vi "configuration UI.vi"() -> ()   [LabVIEW 2013, in "user tag bus module editor node.lvclass"]
uses:
  user tag bus module editor node.lvclass
  <vilib>/CEF_TreeControl/Node/NodeRef.ctl
  <vilib>/CEF_TreeControl/Node/NISE_CEF_Node.lvclass
  <vilib>/NI/AMC/Message Queue.ctl
  <vilib>/NI/AMC/Message.ctl
  <vilib>/NI/Tools/Keyed Array/KeyedArray.ctl
  <vilib>/CEF_TreeControl/Node/UserEventRef.ctl
  <vilib>/CEF_TreeControl/Controls/EventCluster.ctl
  module/configuration/user tag bus module configuration.lvclass
  module/configuration/control module configuration.ctl
  <vilib>/NI/Tag Bus Module Framework/channel/TBM channel.lvclass
  module/configuration/gains.ctl
  module/configuration/state module configuration.ctl
  user tag bus module editor node.lvclass/user tag bus module editor node.ctl
  <vilib>/NI/Tag Bus Module Framework/root configuration/TBM configuration.lvclass/TBM configuration.ctl
  Configuration Editor/Classes/Engine Parent/Engine Parent Editor Node.lvclass
  module/configuration/user tag bus module configuration.lvclass/user tag bus module configuration.ctl
  Read sort_.vi
  module/configuration/Read state module configuration.vi
  Write sort_.vi
  <vilib>/NI/Tag Bus Module Framework/root configuration/Read instance name.vi
  Configuration Editor/Classes/Module editor node/Read Module Configuration.vi
  <vilib>/NI/Tag Bus Module Framework/root configuration/create GUID.vi
  <vilib>/NI/Tag Bus Module Framework/module configuration/TBM module configuration.lvclass
  <vilib>/CEF_TreeControl/NISE_CEF_TreeControl.lvlib
  <vilib>/NI/Tools/Keyed Array/Tools_KeyedArray.lvlib
  <vilib>/NI/AMC/AMC.lvlib
panel:
  in  "Tab Control":T1(tab)
  in  "delete":bool
  in  "add":bool
  in  "Result Tag":u16(ring)
  in  "PV Tag":u16(ring)
  in  "Setpoint Tag":u16(ring)
  in  "Functions":i32(listbox)
  in  "Function Name":string
  in  "Lower Limit":dbl=-100.0
  in  "Upper Limit":dbl=100.0
  in  "Ki":dbl
  in  "Kd":dbl
  in  "Kp":dbl
  in  "Output Tag":u16(ring)
  in  "Input Tag":u16(ring)
  in  "Initial State":u8
  in  "user event":T2
  in  "main queue":T3
  in  "node ref":T4
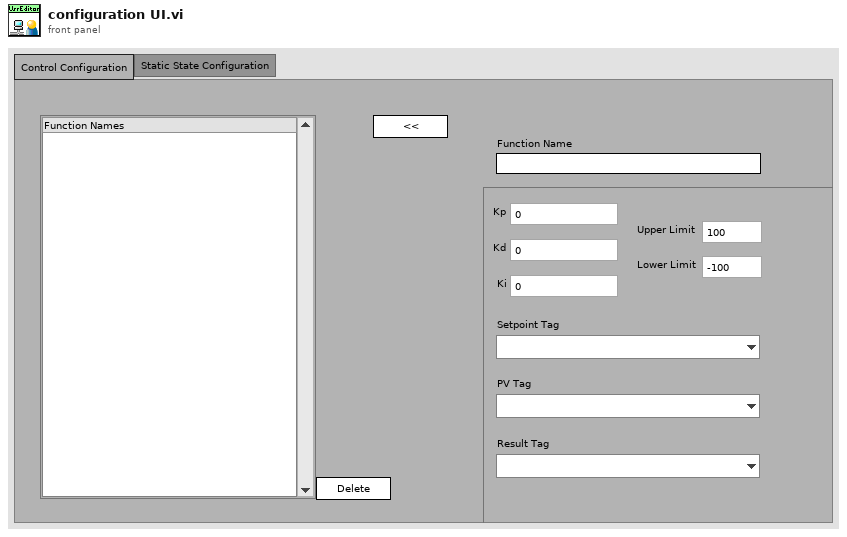
[diagram p1: front panel]
types:
  T1 = enum32{"Control Configuration", "Static State Configuration"}
  T2 = typedef "NISE_CEF_Node.lvclass/UserEventRef.ctl" = refnum<user-event>
  T3 = typedef "AMC.lvlib/Message Queue.ctl" = refnum<queue>
  T4 = typedef "NISE_CEF_Node.lvclass/NodeRef.ctl" = refnum<data-value>
  T5 = typedef "user tag bus module configuration.lvclass/state module configuration.ctl" = cluster{"fixed input":refnum<class "TBM channel.lvclass">, "fixed output":refnum<class "TBM channel.lvclass">, "initial state":u8}
  T6 = typedef "user tag bus module configuration.lvclass/control module configuration.ctl" = cluster{"name":string, "setpoint":refnum<class "TBM channel.lvclass">, "process variable":refnum<class "TBM channel.lvclass">, "output":refnum<class "TBM channel.lvclass">, "gains":T7, "output range":cluster{"output high":dbl, "output low":dbl}}
  T7 = typedef "user tag bus module configuration.lvclass/gains.ctl" = cluster{"Kp":dbl, "Ki":dbl, "Kd":dbl}
  T8 = typedef "NISE_CEF_TreeControl.lvlib/EventCluster.ctl" = cluster{"command":string, "data":string}
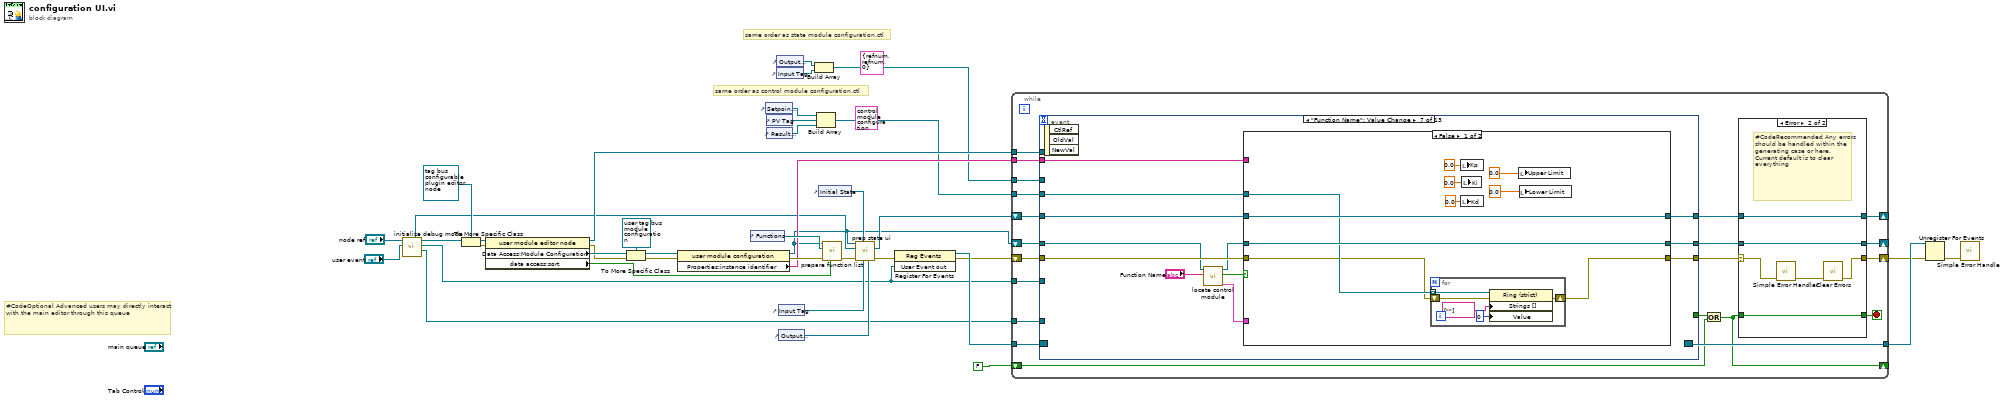
[diagram p0: block diagram]
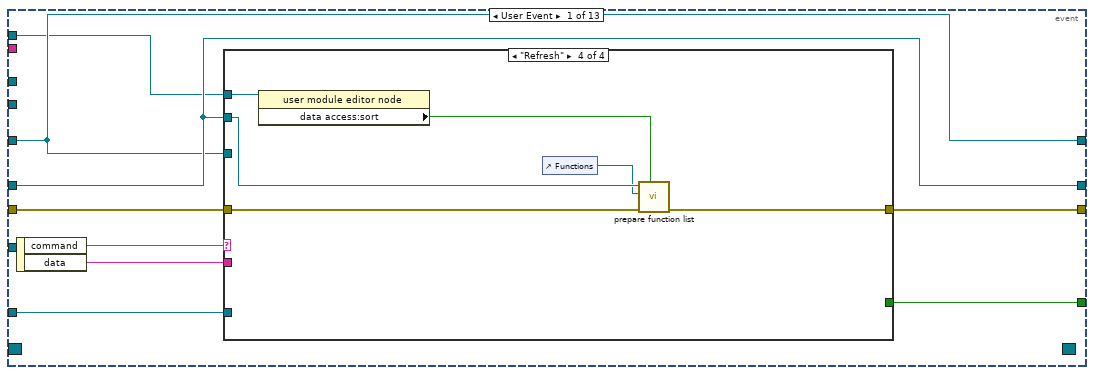
[diagram p3: hidden frame]
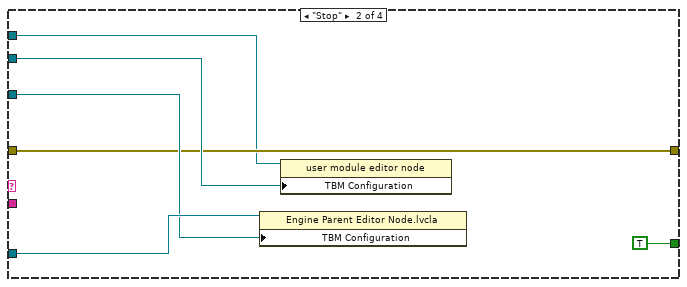
[diagram p5: hidden frame]
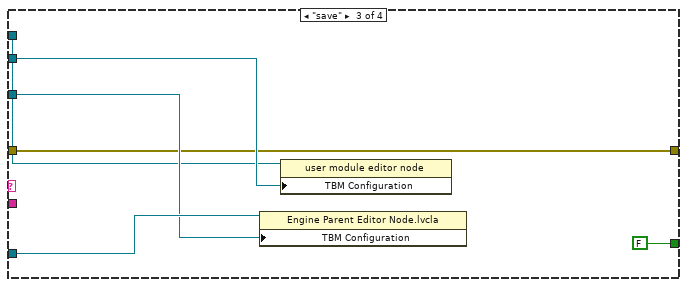
[diagram p6: hidden frame]
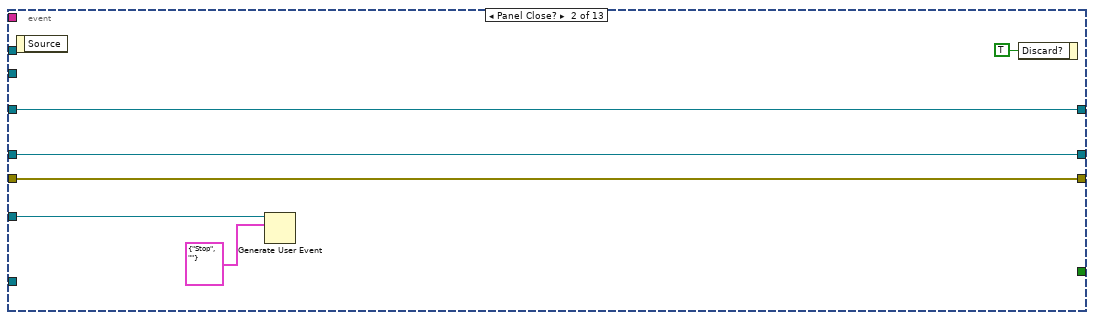
[diagram p7: hidden frame]
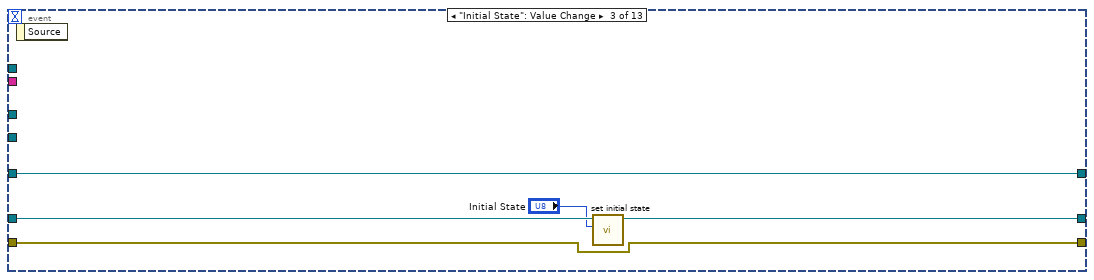
[diagram p8: hidden frame]
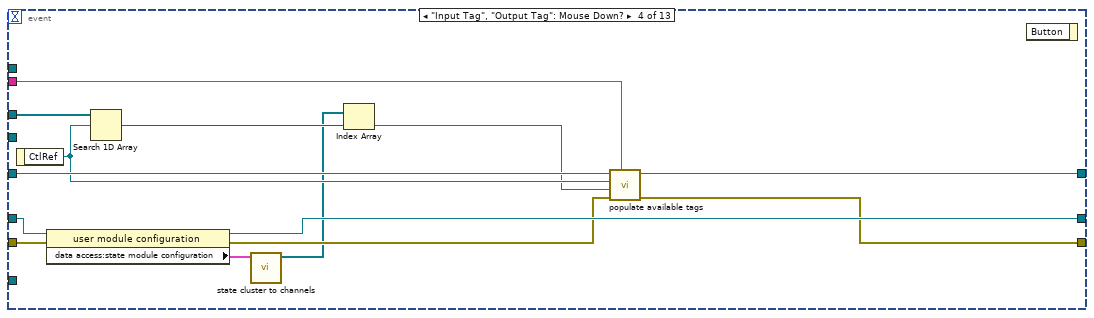
[diagram p9: hidden frame]
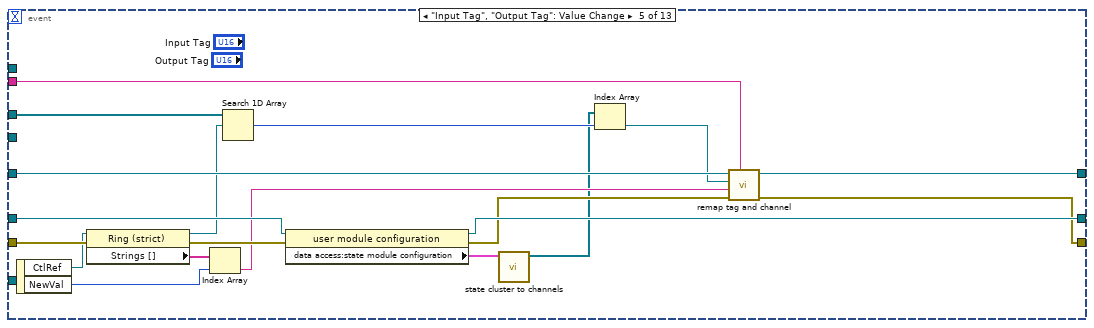
[diagram p10: hidden frame]
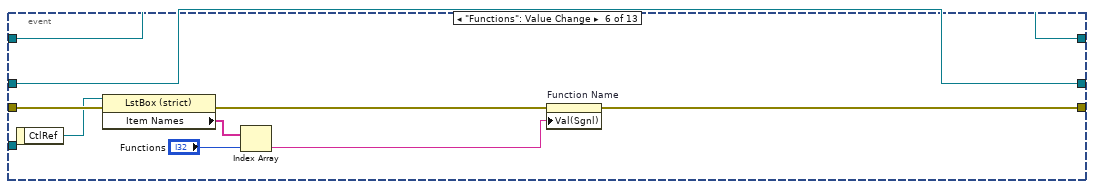
[diagram p11: hidden frame]
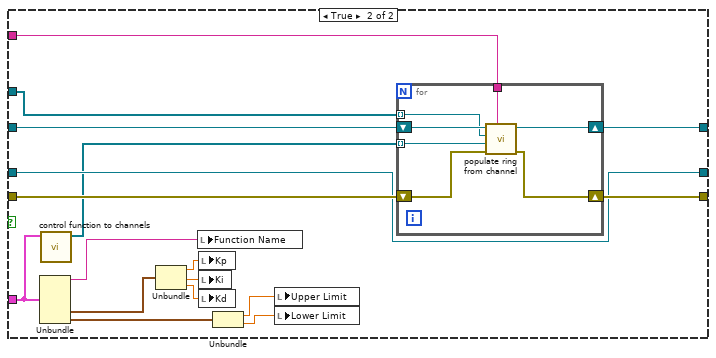
[diagram p12: hidden frame]
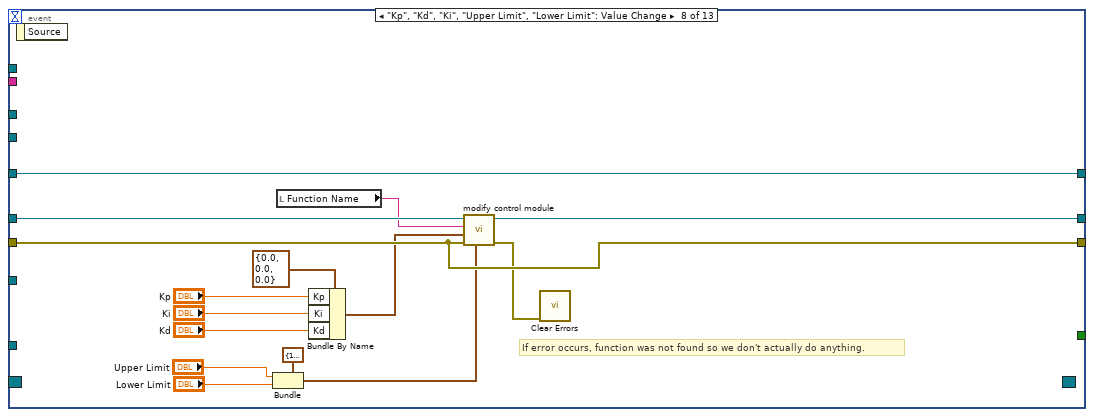
[diagram p13: hidden frame]
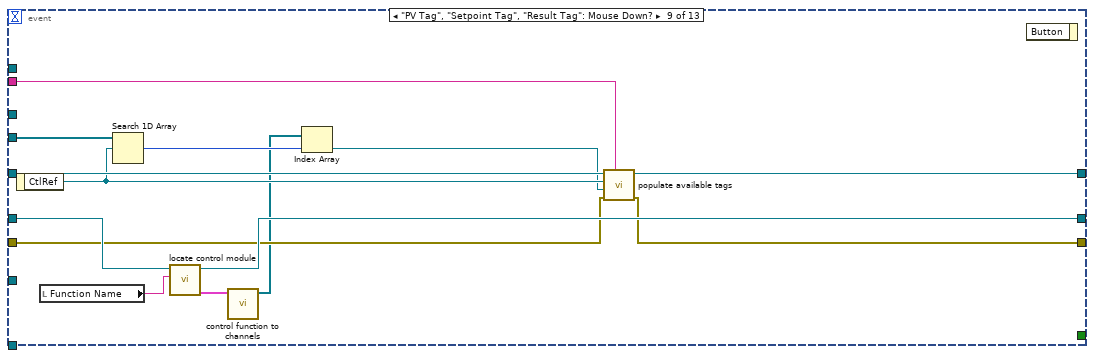
[diagram p14: hidden frame]
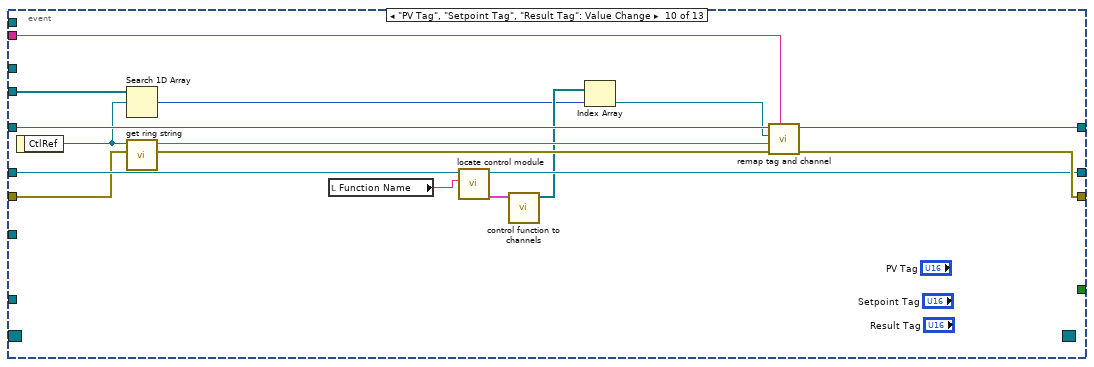
[diagram p15: hidden frame]
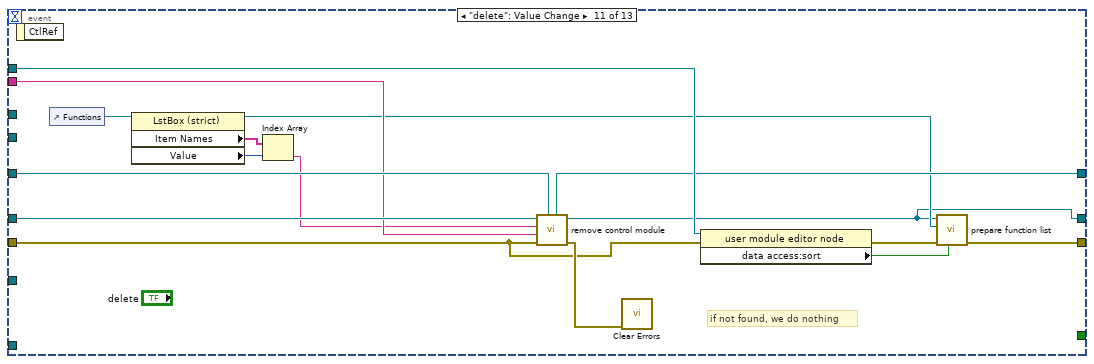
[diagram p16: hidden frame]
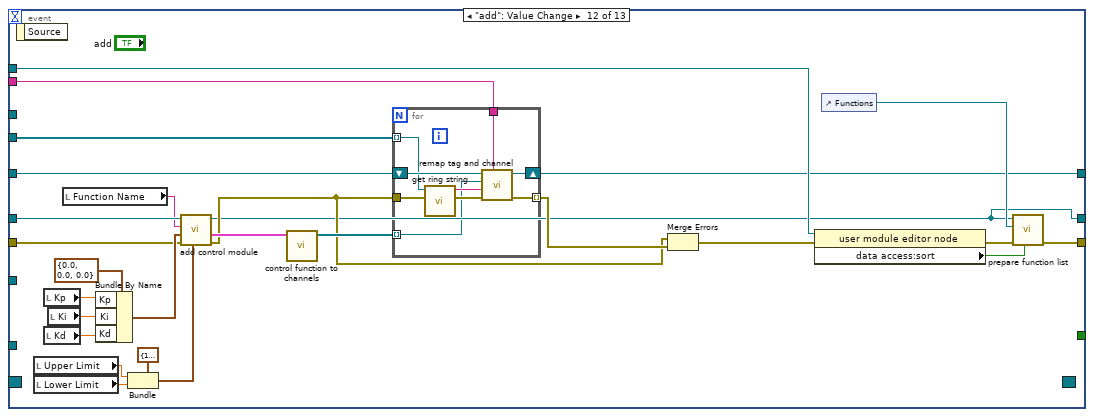
[diagram p17: hidden frame]
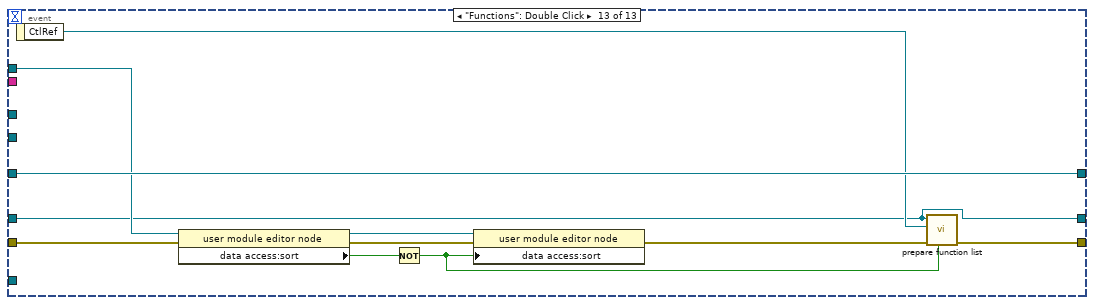
[diagram p18: hidden frame]
diagram:
  (unwired) T5 {"fixed input"=refnum, "fixed output"=refnum, "initial state"=0} ("state module configuration")
  (unwired) T6 {"name"="", "setpoint"=refnum, "process variable"=refnum, "output"=refnum, "gains"={"Kp"=0.0, "Ki"=0.0, "Kd"=0.0}, "output range"={"output high"=100.0, "output low"=-100.0}} ("control module configuration")
  # "same order as control module configuration.ctl"
  # "same order as state module configuration.ctl"
  # "#CodeOptional Advanced users may directly interact with the main editor through this queue"
  n1 = call "initialize debug mode.vi"("User Event in"="user event", "editor node in"="node ref") -> ("engine"=w11:refnum<data-value>, "User Event out"=w4:T2, "editor node out"=w14:T4, "Engine Configuration"=w10:refnum<class "engine configuration.lvclass">)  [unwired: 6 in]
  n2 = To More Specific Class(target class=refnum<data-value> refnum ("data value reference"), reference=w14) -> (specific class reference=w32:refnum<data-value>, error out=w31:errorcluster)  [unwired: 1 in]
  n3 = property class="user module editor node"(reference=w32, error in=w31) -> (reference out=w16:refnum<data-value>, error out=w26:errorcluster, "Data Access:Module Configuration"=w30:refnum<class "TBM module configuration.lvclass">, "data access:sort"=w15:bool)
  n4 = To More Specific Class(target class=refnum<class "user tag bus module configuration.lvclass"> refnum ("user module configuration"), reference=w30, error in=w26) -> (specific class reference=w24:refnum<class "user tag bus module configuration.lvclass">, error out=w28:errorcluster)
  n5 = property class="user module configuration"(reference=w24, error in=w28) -> (reference out=w3:refnum<class "user tag bus module configuration.lvclass">, error out=w25:errorcluster, "Properties:instance identifier"=w23:string)
  n6 = control-ref of="Functions"() -> (w27:refnum<vi>)
  n7 = control-ref of="Setpoint Tag"() -> (w2:refnum<vi>)
  n8 = control-ref of="PV Tag"() -> (w7:refnum<vi>)
  n9 = control-ref of="Result Tag"() -> (w1:refnum<vi>)
  n10 = control-ref of="Output Tag"() -> (w8:refnum<vi>)
  n11 = control-ref of="Input Tag"() -> (w9:refnum<vi>)
  n12 = control-ref of="Input Tag"() -> (w19:refnum<vi>)
  n13 = control-ref of="Output Tag"() -> (w18:refnum<vi>)
  n14 = Build Array(w8, w9) -> (w6:refnum<vi>[])
  n15 = Build Array(w2, w7, w1) -> (w5:refnum<vi>[])
  n16 = control-ref of="Initial State"() -> (w20:refnum<vi>)
  n17 = call "prepare function list.vi"("sort?"=w15, "error in"=w25, "Functions listbox"=w27, "configuration in"=w3) -> ("error out"=w21:errorcluster)  [unwired: 5 in]
  n18 = call "prep state ui.vi"("Output Tag"=w18, "Input Tag"=w19, "Initial State"=w20, "error in"=w21, "engine configuration in"=w10, "user tag bus module configuration in"=w3) -> ("error out"=w22:errorcluster, "engine configuration out"=w17:refnum<class "engine configuration.lvclass">)  [unwired: 4 in]
  n19 = register-events(error in=w22, w4) -> (reference out=w39:refnum<event-registration>, error out=w34:errorcluster)  [unwired: 1 in]
  n20 = while {
    tunnel: w39 -> [w60]
    tunnel: [w59] -> w38
    shift-right: [w52] -> w37
    shift-left: w34 -> [w58]
    shift-right: [w54] -> _
    shift-left: FALSE -> [w53]
    shift-right: [w49] -> _
    shift-left: w3 -> [w51]
    shift-right: [w46] -> _
    shift-left: w17 -> [w48]
    tunnel: w23 -> [w45]
    tunnel: w16 -> [w44]
    tunnel: w11 -> [w43]
    tunnel: w6 -> [w42]
    tunnel: w5 -> [w41]
    tunnel: w4 -> [w40]
    stop <- w56 stop-if-true
    n21 = event shown="[6] \"Function Name\": Value Change" {
      selector: w60 -> [_ _ _ _ _ _ _ _ _ _ _ _ _]
      dyn-events: [_ _ _ _ _ _ _ _ _ _ _ _ _] -> w59
      timeout: _ -> [_ _ _ _ _ _ _ _ _ _ _ _ _]
      tunnel: [w77 _ _ _ _ _ _ _ _ _ _ _ _] -> w55
      tunnel: [w78 w104 w108 w119 w134 w143 w159 w216 w224 w245 w261 w290 w309] -> w57
      tunnel: w58 -> [w79 w104 w108 w123 w142 w151 w163 w216 w225 w238 w258 w272 w308]
      tunnel: [w75 w103 w107 w120 w136 w150 w160 w214 w230 w241 w248 w264 w300] -> w50
      tunnel: w51 -> [w75 w103 w109 w121 w137 w150 w158 w217 w231 w242 w263 w282 w300]
      tunnel: w48 -> [w74 w102 w105 w118 w139 w149 w161 w212 w228 w247 w255 w283 w310]
      tunnel: [w74 w102 w105 w122 w135 w149 w162 w212 w227 w246 w254 w284 w310] -> w47
      tunnel: w45 -> [_ _ _ w117 w132 _ w154 _ w226 w244 w253 w285 _]
      tunnel: w44 -> [w73 _ _ _ _ _ _ _ _ _ w256 w286 w304]
      tunnel: w43 -> [w72 _ _ _ _ _ _ _ _ _ _ _ _]
      tunnel: w42 -> [_ _ _ w115 w130 _ _ _ _ _ _ _ _]
      tunnel: w41 -> [_ _ _ _ _ _ w152 _ w222 w237 _ w267 _]
      tunnel: w40 -> [_ w100 _ _ _ _ _ _ _ _ _ _ _]
      event User Event {
        n22 = event-data() -> ("command"=w76:string, "data"=w71:string)  [unwired: 1 in]
        n23 = case shown="\"Refresh\"" w76 {
          tunnel: [_ TRUE FALSE _] -> w77
          tunnel: w72 -> [_ w85 w91 _]
          tunnel: w75 -> [_ w84 w90 w95]
          tunnel: w74 -> [_ w83 w89 _]
          tunnel: w79 -> [w80 w82 w88 w96]
          tunnel: [w80 w82 w88 w97] -> w78
          tunnel: w73 -> [_ w81 w87 w98]
          tunnel: w71 -> [_ _ _ _]
          frame Default {
          }
          frame "Stop" {
            n24 = property class="Engine Parent Editor Node.lvcla"(reference=w85, "TBM Configuration"=w83) -> ()  [unwired: 1 in, 2 out]
            n25 = property class="user module editor node"(reference=w81, "TBM Configuration"=w84) -> ()  [unwired: 1 in, 2 out]
          }
          frame "save" {
            n26 = property class="Engine Parent Editor Node.lvcla"(reference=w91, "TBM Configuration"=w89) -> ()  [unwired: 1 in, 2 out]
            n27 = property class="user module editor node"(reference=w87, "TBM Configuration"=w90) -> ()  [unwired: 1 in, 2 out]
          }
          frame "Refresh" {
            n28 = property class="user module editor node"(reference=w98) -> ("data access:sort"=w94:bool)  [unwired: 1 in, 2 out]
            n29 = control-ref of="Functions"() -> (w93:refnum<vi>)
            n30 = call "prepare function list.vi"("sort?"=w94, "error in"=w96, "Functions listbox"=w93, "configuration in"=w95) -> ("error out"=w97:errorcluster)  [unwired: 5 in]
          }
        }
      }
      event Panel Close? {
        n31 = event-data() -> ()  [unwired: 1 in, 1 out]
        n32 = Generate User Event(user event=w100, event data cluster=T8 {"command"="Stop", "data"=""} ("event data")) -> ()  [unwired: 2 in, 2 out]
        n33 = event-data("Discard?"=TRUE) -> ()  [unwired: 1 in, 1 out]
      }
      event "Initial State": Value Change {
        n34 = event-data() -> ()  [unwired: 1 in, 1 out]
        n35 = call "set initial state.vi"("state module configuration.initial state"="Initial State", "tag bus configurable plugin module configuration in"=w109) -> ("tag bus configurable plugin module configuration out"=w107:refnum<class "user tag bus module configuration.lvclass">)  [unwired: 9 in]
      }
      event "Input Tag", "Output Tag": Mouse Down? {
        n36 = event-data() -> ("CtlRef"=w114:refnum<vi>)  [unwired: 1 in]
        n37 = property class="user module configuration"(reference=w121, error in=w123) -> (reference out=w120:refnum<class "user tag bus module configuration.lvclass">, error out=w116:errorcluster, "data access:state module configuration"=w112:T5)
        n38 = Search 1D Array(1D array=w115, element=w114) -> (index of element=w113:i32)  [unwired: 1 in]
        n39 = call "state cluster to channels.vi"("state module configuration"=w112) -> ("channels"=w111:refnum<class "TBM channel.lvclass">[])  [unwired: 10 in]
        n40 = Index Array(array=w111, index=w113) -> (element=w110:refnum<class "TBM channel.lvclass">)
        n41 = call "populate available tags.vi"("instance id"=w117, "error in"=w116, "channel"=w110, "CtlRef"=w114, "engine configuration in"=w118) -> ("error out"=w119:errorcluster, "engine configuration out"=w122:refnum<class "engine configuration.lvclass">)  [unwired: 5 in]
        n42 = event-data() -> ()  [unwired: 2 in, 1 out]
      }
      event "Input Tag", "Output Tag": Value Change {
        n43 = event-data() -> ("CtlRef"=w141:refnum<vi>, "NewVal"=w128:u16)  [unwired: 1 in]
        n44 = property on="Property Node" class="Ring (strict)"(reference=w141, error in=w142) -> (reference out=w129:refnum<vi>, error out=w138:errorcluster, "Strings []"=w140:string[])
        n45 = Index Array(array=w140, index=w128) -> (element=w131:string)
        n46 = Search 1D Array(1D array=w130, element=w129) -> (index of element=w126:i32)  [unwired: 1 in]
        n47 = property class="user module configuration"(reference=w137, error in=w138) -> (reference out=w136:refnum<class "user tag bus module configuration.lvclass">, error out=w133:errorcluster, "data access:state module configuration"=w127:T5)
        n48 = call "state cluster to channels.vi"("state module configuration"=w127) -> ("channels"=w125:refnum<class "TBM channel.lvclass">[])  [unwired: 10 in]
        n49 = Index Array(array=w125, index=w126) -> (element=w124:refnum<class "TBM channel.lvclass">)
        n50 = call "remap tag and channel.vi"("instance id"=w132, "error in"=w133, "tag name"=w131, "channel"=w124, "engine configuration in"=w139) -> ("error out"=w134:errorcluster, "engine configuration out"=w135:refnum<class "engine configuration.lvclass">)  [unwired: 5 in]
      }
      event "Functions": Value Change {
        n51 = event-data() -> ("CtlRef"=w148:refnum<vi>)  [unwired: 1 in]
        n52 = property class="LstBox (strict)"(reference=w148, error in=w151) -> (error out=w144:errorcluster, "Item Names"=w147:string[])  [unwired: 1 out]
        n53 = Index Array(array=w147, index="Functions") -> (element=w145:string)
        n54 = property on="Function Name" class="Str"(error in=w144, "Val(Sgnl)"=w145) -> (error out=w143:errorcluster)  [unwired: 1 in, 1 out]
      }
      event "Function Name": Value Change {
        n55 = event-data() -> ()  [unwired: 1 in, 3 out]
        n56 = call "locate control module.vi"("name"="Function Name", "user module configuration in"=w158) -> ("module duplicate"=w155:T6, "found"=w156:bool, "user module configuration out"=w157:refnum<class "user tag bus module configuration.lvclass">)  [unwired: 6 in, 1 out]
        n57 = case shown="False" w156 {
          tunnel: [w173 w187] -> w162
          tunnel: w161 -> [w173 w185]
          tunnel: w157 -> [w172 w182]
          tunnel: [w172 w182] -> w160
          tunnel: w163 -> [w170 w184]
          tunnel: [w169 w183] -> w159
          tunnel: w155 -> [_ w181]
          tunnel: w154 -> [_ w186]
          tunnel: w152 -> [w171 w180]
          frame False {
            n58 = for {
              shift-right: [w178] -> w169
              shift-left: w170 -> [w177]
              tunnel: w171 -> [w175] mode=indexing
              n59 = property on="Property Node" class="Ring (strict)"(reference=w175, error in=w177, "Strings []"=string[] [""], "Value"=u16 0) -> (error out=w178:errorcluster)  [unwired: 1 out]
            }
            n60 = local write "Kp"(0.0 ("Kp")) -> ()
            n61 = local write "Kd"(0.0 ("Kp")) -> ()
            n62 = local write "Ki"(0.0 ("Kp")) -> ()
            n63 = local write "Upper Limit"(0.0 ("Kp")) -> ()
            n64 = local write "Lower Limit"(0.0 ("Kp")) -> ()
          }
          frame True {
            n65 = Unbundle(w181) -> ("name"=w188:string, "gains"=w195:T7, "output range"=w194:cluster{"output high":dbl, "output low":dbl})  [unwired: 3 out]
            n66 = call "control function to channels.vi"("control module configuration"=w181) -> ("channels"=w179:refnum<class "TBM channel.lvclass">[])  [unwired: 10 in]
            n67 = Unbundle(w195) -> ("Kp"=w189:dbl, "Ki"=w190:dbl, "Kd"=w191:dbl)
            n68 = local write "Function Name"(w188) -> ()
            n69 = local write "Kp"(w189) -> ()
            n70 = local write "Ki"(w190) -> ()
            n71 = local write "Kd"(w191) -> ()
            n72 = Unbundle(w194) -> ("output high"=w192:dbl, "output low"=w193:dbl)
            n73 = local write "Upper Limit"(w192) -> ()
            n74 = local write "Lower Limit"(w193) -> ()
            n75 = for {
              tunnel: w186 -> [w201]
              shift-right: [w202] -> w187
              shift-left: w185 -> [w200]
              shift-right: [w198] -> w183
              shift-left: w184 -> [w199]
              tunnel: w180 -> [w197] mode=indexing
              tunnel: w179 -> [w196] mode=indexing
              n76 = call "populate ring from channel.vi"("instance id"=w201, "error in"=w199, "channel"=w196, "ring"=w197, "engine configuration in"=w200) -> ("error out"=w198:errorcluster, "engine configuration out"=w202:refnum<class "engine configuration.lvclass">)  [unwired: 4 in, 1 out]
            }
          }
        }
      }
      event "Kp", "Kd", "Ki", "Upper Limit", "Lower Limit": Value Change {
        # "If error occurs, function was not found so we don't actually do anything."
        n77 = event-data() -> ()  [unwired: 1 in, 1 out]
        n78 = Bundle(cluster=cluster{"output high":dbl, "output low":dbl} {"output high"=100.0, "output low"=-100.0} ("output range"), "output high"="Upper Limit", "output low"="Lower Limit") -> (w208:cluster{"output high":dbl, "output low":dbl})
        n79 = local read "Function Name"() -> (w213:string)
        n80 = Bundle By Name(cluster=T7 {"Kp"=0.0, "Ki"=0.0, "Kd"=0.0} ("gains"), "Kp"="Kp", "Ki"="Ki", "Kd"="Kd") -> (w203:T7)
        n81 = call "modify control module.vi"("output range"=w208, "error in"=w216, "gains"=w203, "name"=w213, "user module configuration in"=w217) -> ("error out"=w215:errorcluster, "user module configuration out"=w214:refnum<class "user tag bus module configuration.lvclass">)  [unwired: 5 in]
        n82 = call <vilib>:"Clear Errors.vi"("error in (no error)"=w215) -> ()  [unwired: 6 in, 1 out]
      }
      event "PV Tag", "Setpoint Tag", "Result Tag": Mouse Down? {
        n83 = event-data() -> ("CtlRef"=w221:refnum<vi>)  [unwired: 1 in]
        n84 = local read "Function Name"() -> (w229:string)
        n85 = Search 1D Array(1D array=w222, element=w221) -> (index of element=w220:i32)  [unwired: 1 in]
        n86 = call "locate control module.vi"("name"=w229, "user module configuration in"=w231) -> ("module duplicate"=w223:T6, "user module configuration out"=w230:refnum<class "user tag bus module configuration.lvclass">)  [unwired: 6 in, 2 out]
        n87 = call "control function to channels.vi"("control module configuration"=w223) -> ("channels"=w219:refnum<class "TBM channel.lvclass">[])  [unwired: 10 in]
        n88 = Index Array(array=w219, index=w220) -> (element=w218:refnum<class "TBM channel.lvclass">)
        n89 = call "populate available tags.vi"("instance id"=w226, "error in"=w225, "channel"=w218, "CtlRef"=w221, "engine configuration in"=w228) -> ("error out"=w224:errorcluster, "engine configuration out"=w227:refnum<class "engine configuration.lvclass">)  [unwired: 5 in]
        n90 = event-data() -> ()  [unwired: 2 in, 1 out]
      }
      event "PV Tag", "Setpoint Tag", "Result Tag": Value Change {
        n91 = event-data() -> ("CtlRef"=w236:refnum<vi>)  [unwired: 1 in]
        n92 = Search 1D Array(1D array=w237, element=w236) -> (index of element=w233:i32)  [unwired: 1 in]
        n93 = call "get ring string.vi"("error in"=w238, "Ring in"=w236) -> ("error out"=w239:errorcluster, "String"=w240:string)  [unwired: 8 in]
        n94 = local read "Function Name"() -> (w243:string)
        n95 = call "locate control module.vi"("name"=w243, "user module configuration in"=w242) -> ("module duplicate"=w235:T6, "user module configuration out"=w241:refnum<class "user tag bus module configuration.lvclass">)  [unwired: 6 in, 2 out]
        n96 = call "control function to channels.vi"("control module configuration"=w235) -> ("channels"=w234:refnum<class "TBM channel.lvclass">[])  [unwired: 10 in]
        n97 = Index Array(array=w234, index=w233) -> (element=w232:refnum<class "TBM channel.lvclass">)
        n98 = call "remap tag and channel.vi"("instance id"=w244, "error in"=w239, "tag name"=w240, "channel"=w232, "engine configuration in"=w247) -> ("error out"=w245:errorcluster, "engine configuration out"=w246:refnum<class "engine configuration.lvclass">)  [unwired: 5 in]
      }
      event "delete": Value Change {
        # "if not found, we do nothing"
        n99 = event-data() -> ()  [unwired: 1 in, 1 out]
        n100 = control-ref of="Functions"() -> (w257:refnum<vi>)
        n101 = property class="LstBox (strict)"(reference=w257) -> (reference out=w252:refnum<vi>, "Item Names"=w251:string[], "Value"=w250:i32)  [unwired: 1 in, 1 out]
        n102 = Index Array(array=w251, index=w250) -> (element=w249:string)
        n103 = call "remove control module.vi"("engine in"=w255, "error in"=w258, "owner id"=w253, "name"=w249, "user module configuration in"=w263) -> ("error out"=w262:errorcluster, "user module configuration out"=w248:refnum<class "user tag bus module configuration.lvclass">, "engine out"=w254:refnum<class "engine configuration.lvclass">)  [unwired: 4 in]
        n104 = call <vilib>:"Clear Errors.vi"("error in (no error)"=w262) -> ()  [unwired: 6 in, 1 out]
        n105 = property class="user module editor node"(reference=w256, error in=w258) -> (error out=w260:errorcluster, "data access:sort"=w259:bool)  [unwired: 1 out]
        n106 = call "prepare function list.vi"("sort?"=w259, "error in"=w260, "Functions listbox"=w252, "configuration in"=w248) -> ("error out"=w261:errorcluster)  [unwired: 5 in]
      }
      event "add": Value Change {
        n107 = event-data() -> ()  [unwired: 1 in, 1 out]
        n108 = local read "Upper Limit"() -> (w281:dbl)
        n109 = local read "Lower Limit"() -> (w280:dbl)
        n110 = local read "Kp"() -> (w275:dbl)
        n111 = local read "Kd"() -> (w277:dbl)
        n112 = local read "Ki"() -> (w276:dbl)
        n113 = local read "Function Name"() -> (w271:string)
        n114 = Bundle By Name(cluster=T7 {"Kp"=0.0, "Ki"=0.0, "Kd"=0.0} ("gains"), "Kp"=w275, "Ki"=w276, "Kd"=w277) -> (w273:T7)
        n115 = Bundle(cluster=cluster{"output high":dbl, "output low":dbl} {"output high"=100.0, "output low"=-100.0} ("output range"), "output high"=w281, "output low"=w280) -> (w278:cluster{"output high":dbl, "output low":dbl})
        n116 = call "add control module.vi"("output range"=w278, "error in"=w272, "gains"=w273, "name"=w271, "user module configuration in"=w282) -> ("error out"=w265:errorcluster, "generated control module"=w269:T6, "user module configuration out"=w264:refnum<class "user tag bus module configuration.lvclass">)  [unwired: 3 in, 1 out]
        n117 = call "control function to channels.vi"("control module configuration"=w269) -> ("channels"=w268:refnum<class "TBM channel.lvclass">[])  [unwired: 10 in]
        n118 = for {
          tunnel: w285 -> [w299]
          shift-right: [w298] -> w284
          shift-left: w283 -> [w297]
          tunnel: w268 -> [w292] mode=indexing
          tunnel: w267 -> [w291] mode=indexing
          tunnel: w265 -> [w294]
          tunnel: [w293] -> w270 mode=indexing
          n119 = call "get ring string.vi"("error in"=w294, "Ring in"=w291) -> ("error out"=w296:errorcluster, "String"=w295:string)  [unwired: 8 in]
          n120 = call "remap tag and channel.vi"("instance id"=w299, "error in"=w296, "tag name"=w295, "channel"=w292, "engine configuration in"=w297) -> ("error out"=w293:errorcluster, "engine configuration out"=w298:refnum<class "engine configuration.lvclass">)  [unwired: 5 in]
        }
        n121 = Merge Errors(w265, w270) -> (w266:errorcluster)
        n122 = property class="user module editor node"(reference=w286, error in=w266) -> (error out=w289:errorcluster, "data access:sort"=w288:bool)  [unwired: 1 out]
        n123 = control-ref of="Functions"() -> (w287:refnum<vi>)
        n124 = call "prepare function list.vi"("sort?"=w288, "error in"=w289, "Functions listbox"=w287, "configuration in"=w264) -> ("error out"=w290:errorcluster)  [unwired: 5 in]
      }
      event "Functions": Double Click {
        n125 = event-data() -> ("CtlRef"=w307:refnum<vi>)  [unwired: 1 in]
        n126 = property class="user module editor node"(reference=w304, error in=w308) -> (reference out=w303:refnum<data-value>, error out=w305:errorcluster, "data access:sort"=w302:bool)
        n127 = Not(x=w302) -> (.not. x?=w301:bool)
        n128 = property class="user module editor node"(reference=w303, error in=w305, "data access:sort"=w301) -> (error out=w306:errorcluster)  [unwired: 1 out]
        n129 = call "prepare function list.vi"("sort?"=w301, "error in"=w306, "Functions listbox"=w307, "configuration in"=w300) -> ("error out"=w309:errorcluster)  [unwired: 5 in]
      }
    }
    n130 = Or(x=w55, y=w53) -> (x .or. y?=w54:bool)
    n131 = case shown="Error" w57 {
      selector: w57 -> [w63 w69]
      tunnel: [w64 w70] -> w56
      tunnel: w54 -> [w64 w70]
      tunnel: [w63 w67] -> w52
      tunnel: w50 -> [w62 w66]
      tunnel: [w62 w66] -> w49
      tunnel: w47 -> [w61 w65]
      tunnel: [w61 w65] -> w46
      frame No Error {
      }
      frame Error {
        # "#CodeRecommended Any errors should be handled within the generating case or here. Current default is to clear everything"
        n132 = call <vilib>:"Simple Error Handler.vi"("error in (no error)"=w69) -> ("error out"=w68:errorcluster)  [unwired: 4 in, 4 out]
        n133 = call <vilib>:"Clear Errors.vi"("error in (no error)"=w68) -> ("error out"=w67:errorcluster)  [unwired: 6 in]
      }
    }
  }
  n134 = Unregister For Events(event registration refnum=w38, error in=w37) -> (error out=w33:errorcluster)
  n135 = call <vilib>:"Simple Error Handler.vi"("error in (no error)"=w33) -> ()  [unwired: 4 in, 5 out]
